vi "ParseChoreo.vi"(7 "Overall":cluster{"Time (s)":dbl, "Distance (ft)":dbl}, 11 "FileName":string="C:\\Users\\zwatx\\Documents\\CameraAnalysis\\Chaos.traj") -> (0 "TrajTime":dbl, 1 "dt array":dbl[](array[numeric]), 2 "Trajectory Data":T2(array[cluster]), 3 "Bordeaux Type":T5, 5 "Points out":T3[](array[typedef]))   [LabVIEW 2025]
uses:
  swerve-template/Type Definitions/Data/Robot Velocities.ctl
  Types/Segment Type.ctl
panel:
  in  "?":T4(array[cluster])
  out "Error":bool
  out "ChoreoTrajectory":T6(array[cluster])
  in  "error in (no error)":errorcluster
  out "Full Filename":string
  out "error out":errorcluster
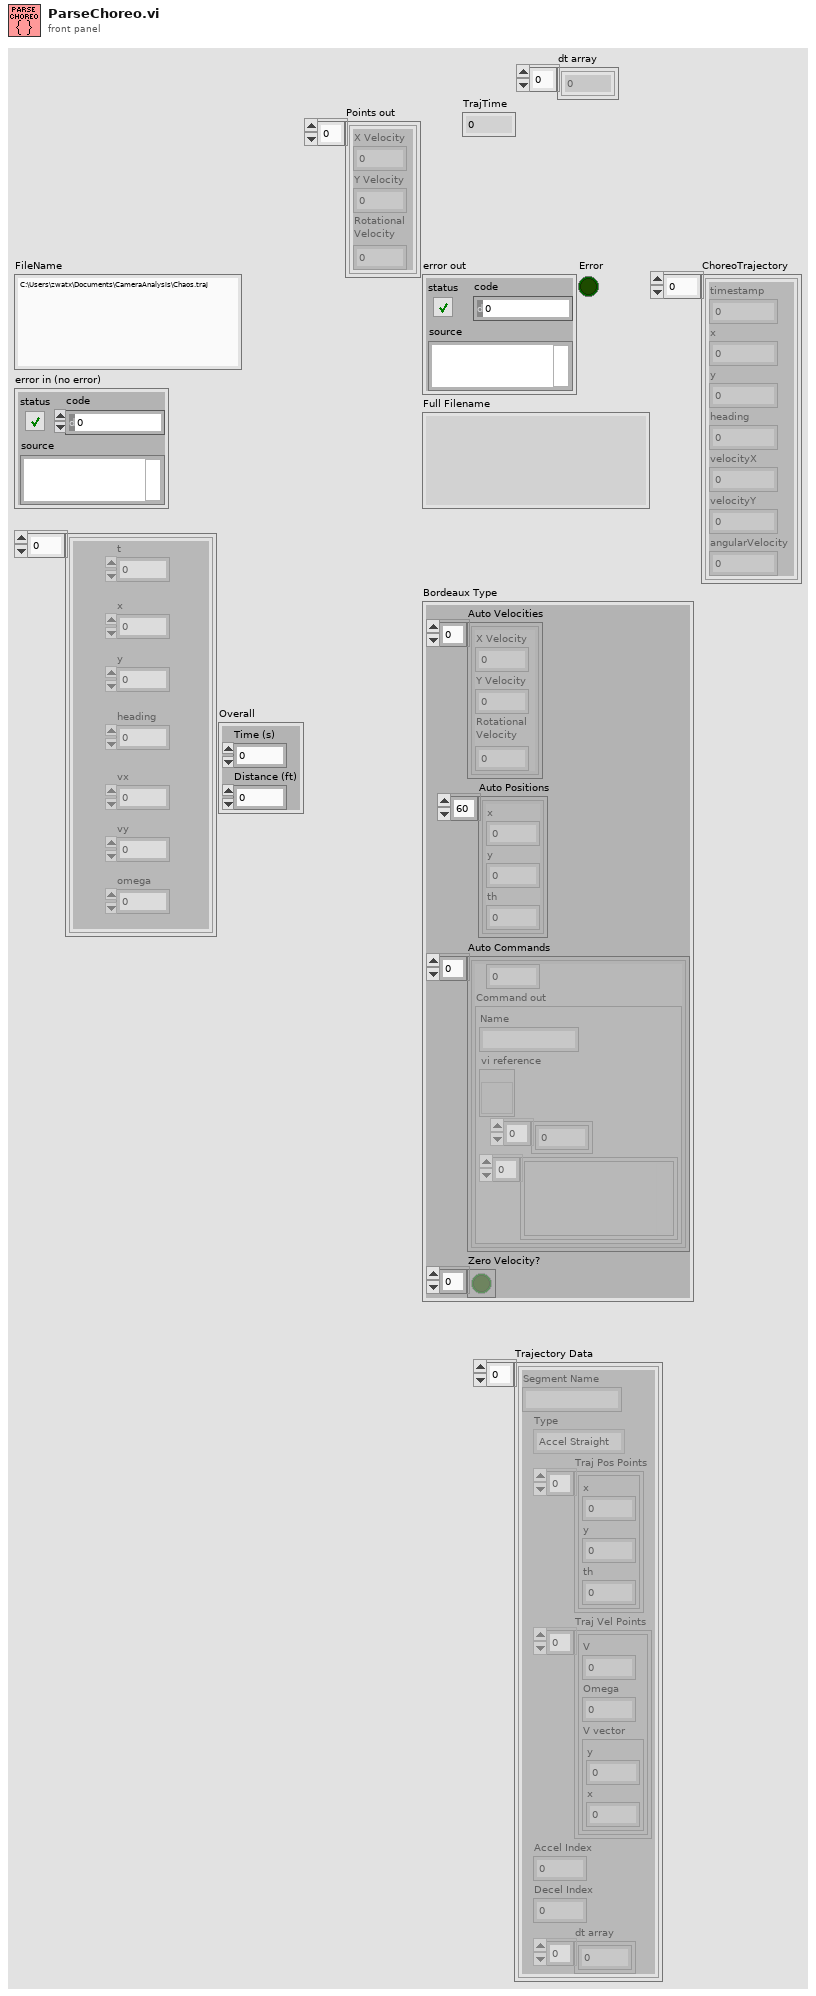
[diagram p1: front panel]
types:
  T1 = typedef "Segment Type.ctl" = enum16{"Accel Straight", "Const Straight", "Blend", "Circle", "Bezier", "Choreo"}
  T2 = cluster{"Segment Name":string, "Type":T1, "Traj Pos Points":cluster{"x":dbl, "y":dbl, "th":dbl}[], "Traj Vel Points":cluster{"V":dbl, "Omega":dbl, "V vector":cluster{"y":dbl, "x":dbl}}[], "Accel Index":i32, "Decel Index":i32, "dt array":dbl[]}[]
  T3 = typedef "Robot Velocities.ctl" = cluster{"X Velocity":dbl, "Y Velocity":dbl, "Rotational \nVelocity":dbl}
  T4 = cluster{"t":dbl, "x":dbl, "y":dbl, "heading":dbl, "vx":dbl, "vy":dbl, "omega":dbl}[]
  T5 = cluster{"Auto Velocities":T3[], "Auto Positions":cluster{"x":dbl, "y":dbl, "th":dbl}[], "Auto Commands":cluster{dbl, "Command out":cluster{"Name":string, "vi reference":refnum<vi>, i32[], variant[]}}[], "Zero Velocity?":bool[]}
  T6 = cluster{"timestamp":dbl, "x":dbl, "y":dbl, "heading":dbl, "velocityX":dbl, "velocityY":dbl, "angularVelocity":dbl}[]
  T7 = enum16{"open", "replace", "create", "open or create", "replace or create", "replace or create with confirmation"}
  T8 = cluster{"timestamp":dbl, "x":dbl, "y":dbl, "heading":dbl, "velocityX":dbl, "velocityY":dbl, "angularVelocity":dbl}
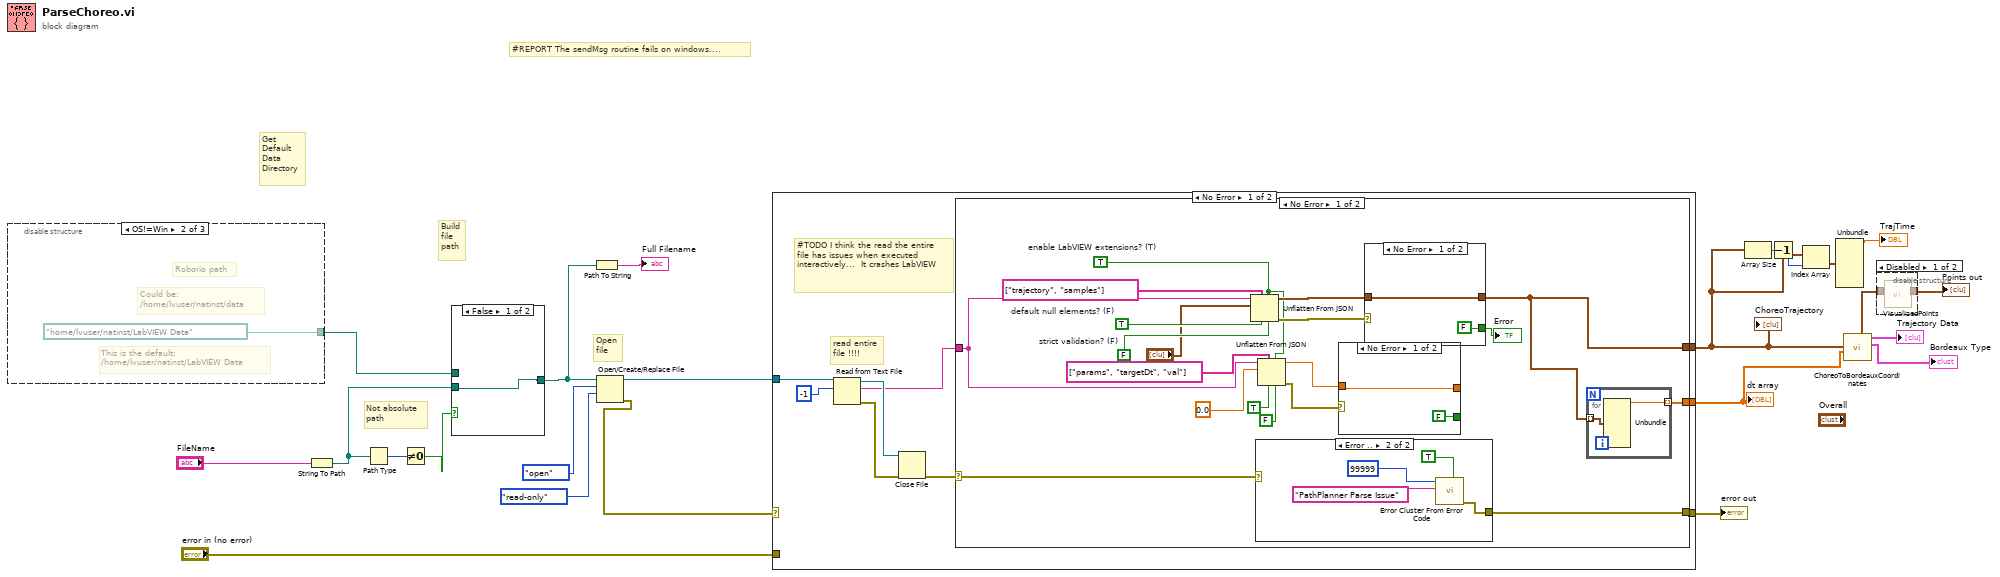
[diagram p0: block diagram]
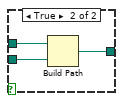
[diagram p3: hidden frame]
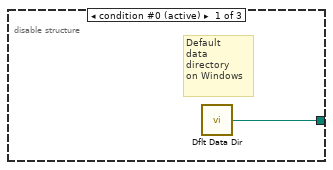
[diagram p4: hidden frame]
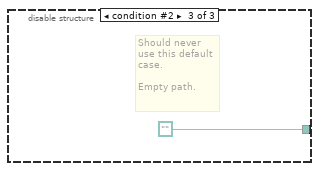
[diagram p5: hidden frame]
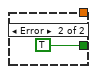
[diagram p6: hidden frame]
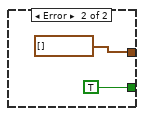
[diagram p7: hidden frame]
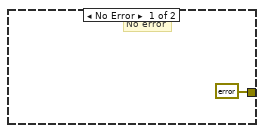
[diagram p8: hidden frame]
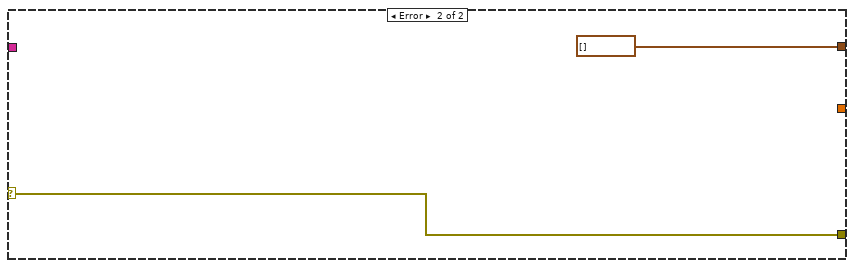
[diagram p9: hidden frame]
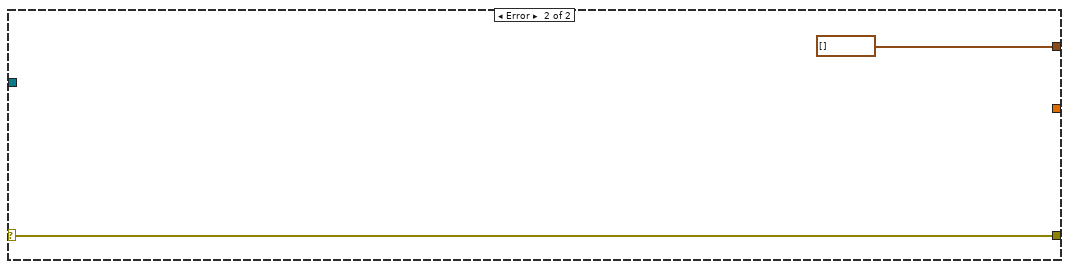
[diagram p10: hidden frame]
diagram:
  # "Not absolute\npath"
  # "#REPORT The sendMsg routine fails on windows...."
  # "Get\nDefault\nData\nDirectory"
  # "Open\nfile"
  # "Build\nfile\npath"
  n1 = disable-structure shown="OS!=Win" {
    disable-tunnel: [w24 path "/home/lvuser/natinst/LabVIEW Data" path ""] -> w20
    frame condition #0 (active) {
      # "Default\ndata\ndirectory\non Windows"
      n2 = call <vilib>:"Dflt Data Dir.vi"() -> ("App:Default Data Directory"=w24:path)
    }
    frame condition #1 {
      # "This is the default:\n/home/lvuser/natinst/LabVIEW Data"
      # "Could be:\n/home/lvuser/natinst/data"
      # "Roborio path"
    }
    frame condition #2 {
      # "Should never\nuse this default\ncase.\n\nEmpty path."
    }
  }
  n3 = String To Path(string="FileName") -> (path=w19:path)
  n4 = Path Type(1:w19) -> (0:w18:i16)
  n5 = Not Equal To 0?(x=w18) -> (x != 0?=w17:bool)
  n6 = case shown="False" w17 {
    tunnel: [w27 w30] -> w14
    tunnel: w20 -> [_ w29]
    tunnel: w19 -> [w27 w28]
    frame False {
    }
    frame True {
      n7 = Build Path(base path=w29, name or relative path=w28) -> (appended path=w30:path)
    }
  }
  n8 = Path To String(path=w14) -> (string=→"Full Filename":string)
  n9 = Open/Create/Replace File(file path (use dialog)=w14, operation (0:open)=T7."open", access (0:read/write)=enum16{"read/write", "read-only", "write-only"}."read-only") -> (refnum out=w15:refnum<file>, error out=w21:errorcluster)  [unwired: 3 in, 1 out]
  n10 = case shown="No Error" w21 {
    selector: w21 -> [_ w76]
    tunnel: w15 -> [w38 _]
    tunnel: [w33 w76] -> w11
    tunnel: "error in (no error)" -> [_ _]
    tunnel: [w32 T6 [] ("ChoreoTrajectory")] -> w8
    tunnel: [w31 _] -> w2
    frame No Error {
      # "#TODO I think the read the entire\nfile has issues when executed\ninteractively...  It crashes LabVIEW"
      # "read entire\nfile !!!!"
      n11 = Read from Text File(file (use dialog)=w38, count=-1) -> (refnum out=w37:refnum<file>, text=w36:string, error out=w35:errorcluster)  [unwired: 2 in, 1 out]
      n12 = Close File(refnum=w37, error in=w35) -> (error out=w34:errorcluster)  [unwired: 1 out]
      n13 = case shown="No Error" w34 {
        selector: w34 -> [w50 w74]
        tunnel: w36 -> [w48 _]
        tunnel: [w58 w74] -> w33
        tunnel: [w40 T6 [] ("ChoreoTrajectory")] -> w32
        tunnel: [w41 _] -> w31
        frame No Error {
          w54 = FALSE  # strict validation? (F)
          w55 = TRUE  # default null elements? (F)
          w47 = TRUE  # enable LabVIEW extensions? (T)
          n14 = Unflatten From JSON(path=string[] ["trajectory", "samples"] ("path 7"), enable LabVIEW extensions? (T)=w47, JSON string=w48, type and defaults="?", default null elements? (F)=w55, strict validation? (F)=w54) -> (value=w56:T4, error out=w57:errorcluster)  [unwired: 1 in]
          n15 = case shown="Error .." w50 {
            tunnel: [errorcluster {"status"=FALSE, "code"=0, "source"=""} ("error out") w69] -> w58
            frame No Error {
              # "No error"
            }
            frame Error {
              n16 = call <vilib>:"Error Cluster From Error Code.vi"("is warning? (False)"=TRUE, "error message (\"\")"="PathPlanner Parse Issue" ("error message (\"\")"), "error code (0)"=99999) -> ("error out"=w69:errorcluster)  [unwired: 6 in]
            }
          }
          n17 = Unflatten From JSON(path=string[] ["params", "targetDt", "val"] ("path 7"), enable LabVIEW extensions? (T)=w47, JSON string=w48, type and defaults=0.0, default null elements? (F)=TRUE, strict validation? (F)=FALSE) -> (value=w43:dbl, error out=w44:errorcluster)  [unwired: 1 in]
          n18 = case shown="No Error" w44 {
            tunnel: w43 -> [w61 _]
            tunnel: [FALSE TRUE] -> _
            tunnel: [w61 _] -> _
            frame No Error {
            }
            frame Error {
            }
          }
          n19 = case shown="No Error" w57 {
            tunnel: w56 -> [w64 _]
            tunnel: [FALSE TRUE] -> w53
            tunnel: [w64 T6 [] ("ChoreoTrajectory 2")] -> w40
            frame No Error {
            }
            frame Error {
            }
          }
          "Error" <- w53
          n20 = for {
            tunnel: w40 -> [w60] mode=indexing
            tunnel: [w59] -> w41 mode=indexing
            n21 = Unbundle(w60) -> ("timestamp"=w59:dbl)  [unwired: 6 out]
          }
        }
        frame Error {
        }
      }
    }
    frame Error {
    }
  }
  "error out" <- w11
  "ChoreoTrajectory" <- w8
  "dt array" <- w2
  n22 = Array Size(array=w8) -> (size(s)=w6:i32)
  n23 = Decrement(x=w6) -> (x-1=w5:i32)
  n24 = Index Array(array=w8, index=w5) -> (element=w9:T8)
  n25 = Unbundle(w9) -> ("timestamp"=→"TrajTime":dbl)  [unwired: 6 out]
  n26 = call "ChoreoToBordeauxCoordinates.vi"("dt array"=w2, "Choreo Type"=w8) -> ("Bordeaux Type"=→"Bordeaux Type":T5, "Trajectory Data"=→"Trajectory Data":T2, "Points out"=w4:T3[])  [unwired: 7 in]
  n27 = disable-structure shown="Disabled" {
    disable-tunnel: w4 -> [w78 w79]
    disable-tunnel: [w77 w79] -> w3
    frame Disabled {
      n28 = call "VisualizedPoints.vi"("WaypointsOverride"=w78) -> ("WaypointsOverride 2"=w77:cluster{"x":dbl, "y":dbl, "th":dbl}[])  [unwired: 10 in]
    }
    frame Enabled {
    }
  }
  "Points out" <- w3
